vi "Initiate.vi"(8 "error in (no error)":errorcluster, 11 "Keysight44xx in":refnum<class "Keysight44xx.lvclass">) -> (0 "error out":errorcluster, 3 "Keysight44xx out":refnum<class "Keysight44xx.lvclass">)   [LabVIEW 2018, in "SpecAnPlugins.lvlib" / "Keysight44xx.lvclass"]
doc: "This function initiates an acquisition. After calling this function, the spectrum analyzer leaves the idle state. This function does not check the instrument status. The user should call the Acquisition Status function to determine when the acquisition is complete."
uses:
  Keysight44xx.lvclass
  C:/Users/ico/Documents/Projects/NistPluggableModules/SpecAn/SpecAnPlugins/SpecAnBaseClass/SpecAnBase.lvclass
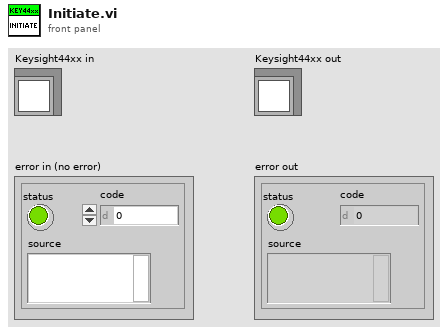
[diagram p1: front panel]
types:
  T1 = typedef "SpecAnPlugins.lvlib/SpecAnBase.lvclass/Acquisition.ctl" = cluster{"Handle":string, "Connected":bool, "Enabled":bool, "SweepModeContinuous":bool, "NumberOfSweeps":i32, "DetectorTypeAuto":bool, "DetectorType":i32, "VerticalScale":i32, "MaximumTime(seconds)":dbl}
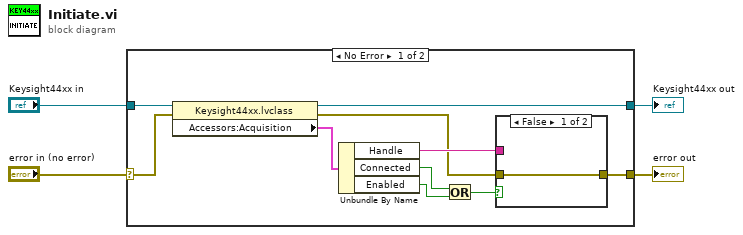
[diagram p0: block diagram]
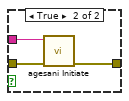
[diagram p2: hidden frame]
diagram:
  n1 = case shown="No Error" "error in (no error)" {
    selector: "error in (no error)" -> [w13 w20]
    tunnel: [w8 w20] -> w3
    tunnel: "Keysight44xx in" -> [w14 w19]
    tunnel: [w11 w19] -> w1
    frame No Error {
      n2 = property class="Keysight44xx.lvclass"(reference=w14, error in=w13) -> (reference out=w11:refnum<class "Keysight44xx.lvclass">, error out=w9:errorcluster, "Accessors:Acquisition"=w12:T1)
      n3 = Unbundle By Name(w12) -> ("Handle"=w10:string, "Connected"=w6:bool, "Enabled"=w5:bool)
      n4 = Or(x=w6, y=w5) -> (x .or. y?=w7:bool)
      n5 = case shown="False" w7 {
        tunnel: w10 -> [_ w18]
        tunnel: w9 -> [w15 w17]
        tunnel: [w15 w16] -> w8
        frame False {
        }
        frame True {
          n6 = call <instrlib>:"agesani Initiate.vi"("error in (no error)"=w17, "instrument handle"=w18) -> ("error out"=w16:errorcluster)  [unwired: 8 in, 1 out]
        }
      }
    }
    frame Error {
    }
  }
  "error out" <- w3
  "Keysight44xx out" <- w1
